vi "Manual_Override.vi"() -> ()   [LabVIEW 2020]
panel:
  out "error out":errorcluster
  in  "error in (no error)":errorcluster
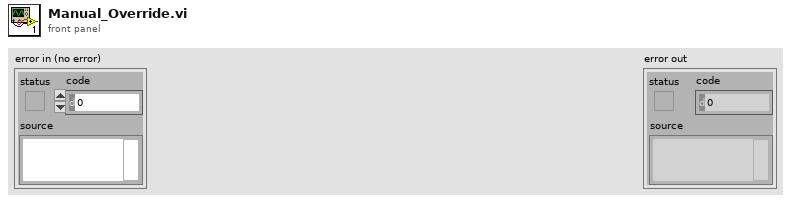
[diagram p1: front panel]
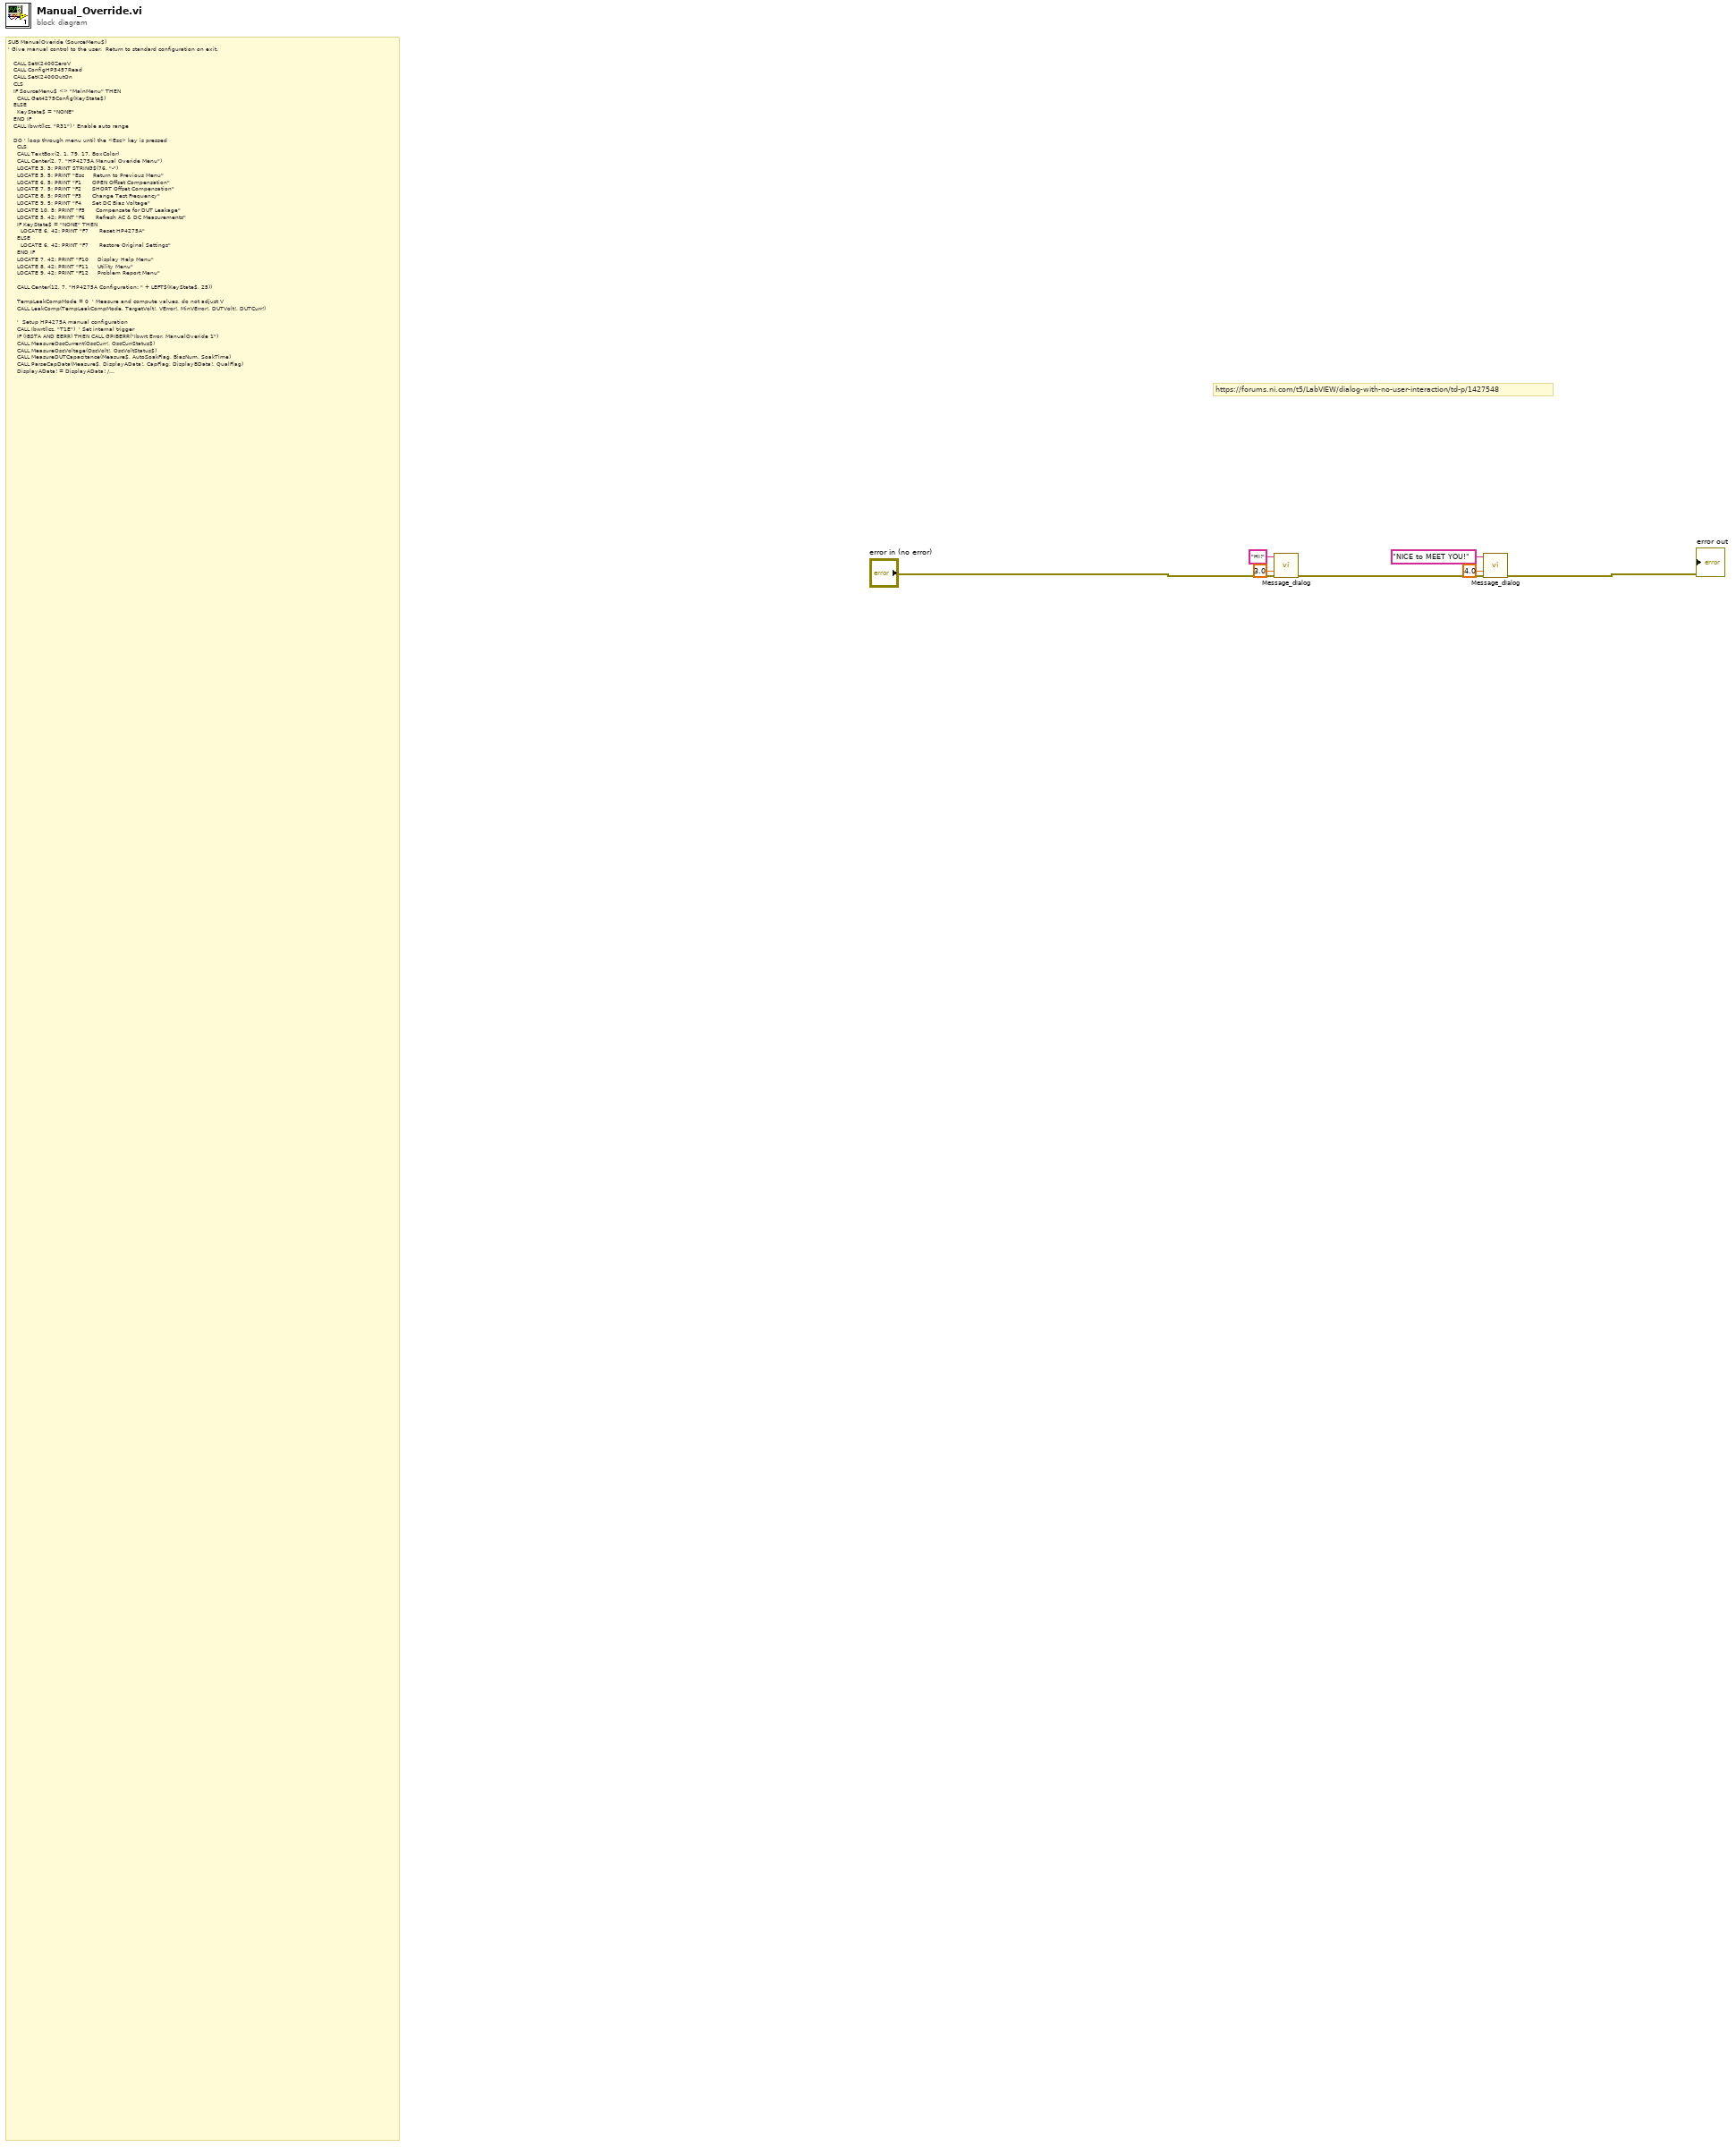
[diagram p0: block diagram]
diagram:
  # "https://forums.ni.com/t5/LabVIEW/dialog-with-no-user-interaction/td-p/1427548"
  # "SUB ManualOveride (SourceMenu$)\n' Give manual control to the user.  Return to standard configuration on exit.\n\n   CALL SetK2400ZeroV\n   CALL ConfigHP3457Read\n   CALL SetK2400OutOn\n   CLS\n   IF SourceMenu$ <> \"MainMenu\" THEN\n     CALL Get4275Config(KeyState$)\n   ELSE\n     KeyState$ = \"NONE\"\n   END IF\n   CALL Ibwrt(lcz, \"R31\") ' Enable auto range\n\n   DO ' loop through menu until the <Esc> key is pressed\n     CLS\n     CALL TextBox(2, 1, 79, 17, BoxColor)\n     CALL Center(2, 7, \"HP4275A Manual Overide Menu\")\n     LOCATE 3, 3: PRINT STRING$(76, \"-\")\n     LOCATE 5, 5: PRINT \"Esc     Return to Previous Menu\"\n     LOCATE 6, 5: PRINT \"F1      OPEN Offset Compensation\"\n     LOCATE 7, 5: PRINT \"F2      SHORT Offset Compensation\"\n     LOCATE 8, 5: PRINT \"F3      Change Test Frequency\"\n     LOCATE 9, 5: PRINT \"F4      Set DC Bias Voltage\"\n     LOCATE 10, 5: PRINT \"F5      Compensate for DUT Leakage\"\n     LOCATE 5, 42: PRINT \"F6      Refresh AC & DC Measurements\"\n     IF KeyState$ = \"NONE\" THEN\n       LOCATE 6, 42: PRINT \"F7      Reset HP4275A\"\n     ELSE\n       LOCATE 6, 42: PRINT \"F7      Restore Original Settings\"\n     END IF\n     LOCATE 7, 42: PRINT \"F10     Display Help Menu\"\n     LOCATE 8, 42: PRINT \"F11     Utility Menu\"\n     LOCATE 9, 42: PRINT \"F12     Problem Report Menu\"\n\n     CALL Center(12, 7, \"HP4275A Configuration: \" + LEFT$(KeyState$, 25))\n\n     TempLeakCompMode = 0  ' Measure and compute values, do not adjust V\n     CALL LeakComp(TempLeakCompMode, TargetVolt!, VError!, MinVError!, DUTVolt!, DUTCurr!)\n\n     '  Setup HP4275A manual configuration\n     CALL Ibwrt(lcz, \"T1E\")  ' Set internal trigger\n     IF (IBSTA AND EERR) THEN CALL GPIBERR(\"Ibwrt Error, ManualOveride 1\")\n     CALL MeasureOscCurrent(OscCurr!, OscCurrStatus$)\n     CALL MeasureOscVoltage(OscVolt!, OscVoltStatus$)\n     CALL MeasureDUTCapacitance(Measure$, AutoSoakFlag, BiasNum, SoakTime)\n     CALL ParseCapData(Measure$, DisplayAData!, CapFlag, DisplayBData!, QualFlag)\n     DisplayAData! = DisplayAData! / 1E+12\n     CALL IBLOC(lcz)\n\n     LOCATE 13, 5\n     PRINT \"Device DC Voltage:  \"; DUTVolt!; \"V\"\n     LOCATE 14, 5\n     PRINT \"Device DC Current:  \"; DUTCurr!; \"A\"\n     LOCATE 15, 5\n     PRINT \"Bias Voltage Error: \"; VError!\n     LOCATE 16, 5\n     PRINT \"Max Voltage Error:  \"; MaxVError!\n\n     LOCATE 13, 47\n     PRINT \"HP4275 Display A: \"; DisplayAData!;\n     LOCATE 14, 47\n     PRINT \"HP4275 Display B: \"; DisplayBData!;\n     LOCATE 15, 47\n     PRINT \"HP4275 Osc V:     \"; OscVolt!; \"V\"\n     LOCATE 16, 47\n     PRINT \"HP4275 Osc I:     \"; OscCurr!; \"A\"\n\n     CALL Center(18, 7, \"Ready\")\n\n     DO\n       Choice$ = INKEY$\n     LOOP WHILE Choice$ = \"\"\n     FOR x! = 1 TO 1000: z = RND: NEXT x!  'Keyboard read delay\n     DO   'Purge keyboard buffer\n       Temp$ = INKEY$\n     LOOP WHILE Temp$ <> \"\"\n\n     '  Convert 2-byte extended code to 1-byte ASCII code\n     Choice$ = RIGHT$(Choice$, 1)\n     SELECT CASE Choice$\n       CASE CHR$(F1)  ' OPEN Offset Compensation\n     CALL SetK2400ZeroV\n     CALL Delay(100)\n     CALL CalibrateOpen(TestLevel!, Flag, AutoSoakFlag)\n     CALL IBLOC(lcz)\n       CASE CHR$(F2)  ' SHORT Offset Compensation\n     CALL SetK2400ZeroV\n     CALL Delay(100)\n     CALL CalibrateShort(Flag, AutoSoakFlag)\n     CALL IBLOC(lcz)\n       CASE CHR$(F3)  ' Change Test Frequency\n     CALL SelectFreq(Flag)\n     CALL IBLOC(lcz)\n       CASE CHR$(F4)  ' Set DC Bias Voltage\n     LOCATE 18, 1: PRINT STRING$(76, \" \")\n     IF INSTR(UCASE$(VoltConfig$), \"H\") > 0 THEN\n       VoltMax! = 200!\n       VoltMin! = -200!\n     ELSE\n       VoltMax! = 35!\n       VoltMin! = -35!\n     END IF\n\n     PRINT \"  Enter bias voltage (\"; : PRINT USING \"####.#\"; VoltMin!;\n     PRINT \"V to\"; : PRINT USING \" +###.#\"; VoltMax!;\n     PRINT \"V).  Enter 999 to quit\";\n     INPUT Temp$\n     TempBias! = VAL(Temp$)\n     IF TempBias! <> 999! THEN\n       IF TempBias! > VoltMax! OR TempBias! < VoltMin! THEN\n         CALL SoundEff(2, 1)\n         PRINT\n         PRINT \"  Bias voltage must be between \";\n         PRINT USING \"####.#\"; VoltMin!;\n         PRINT \"V and \";\n         PRINT USING \"+###.#\"; VoltMax!;\n         PRINT \"V.\"\n         SLEEP 4: CALL SoundEff(2, 1)\n       ELSE\n         CALL SetK2400Voltage(TempBias!)\n         CALL Delay(300)\n         CALL MeasureDUTCurrent(DUTCurr!)\n       END IF\n     END IF\n       CASE CHR$(F5)  ' Compensate for DUT Leakage\n     LOCATE 18, 1: PRINT STRING$(76, \" \")\n     TargetVolt! = TempBias!\n     TempLeakCompMode = 1\n     CALL LeakComp(TempLeakCompMode, TargetVolt!, VError!, MinVError!, DUTVolt!, DUTCurr!)\n       CASE CHR$(F6)   ' Refresh AC & DC Measurements\n     ' Do nothing, measurements are updated every loop\n     LOCATE 18, 1: PRINT STRING$(76, \" \")\n       CASE CHR$(F7)  ' Reset HP4275A or Restore Original Settings\n     LOCATE 18, 1: PRINT STRING$(76, \" \")\n     CALL SetK2400ZeroV\n     IF KeyState$ = \"NONE\" THEN\n       CALL Ibclr(lcz)  ' Reset the HP4275A\n       CALL IBLOC(lcz)\n     ELSE\n       ' Restore original configuration\n       CALL Restore4275Config(KeyState$)\n       CALL Delay(100)\n       CALL Ibwrt(lcz, \"T1E\")  ' Set internal trigger\n       IF (IBSTA AND EERR) THEN CALL GPIBERR(\"Ibwrt Error, ManualOveride 2\")\n     END IF\n     CALL IBLOC(lcz)\n       CASE CHR$(F10)  ' Display Helpfile\n     CALL HelpMenu\n       CASE CHR$(F11)  ' Utility Menu\n     CALL UtilityMenu(SoakTime)\n       CASE CHR$(F12)  ' Problem Report Menu\n     ' Display report menu\n     CALL SelectReportType\n       CASE CHR$(Esc) ' Return to Previous Menu\n     LOCATE 18, 1: PRINT STRING$(76, \" \")\n       CASE ELSE\n     LOCATE 18, 1: PRINT STRING$(76, \" \")\n     LOCATE 18: PRINT \"      Invalid entry; returning to manual menu\"\n     CALL SoundEff(5, 1)\n     SLEEP 2\n     END SELECT\n   LOOP WHILE Choice$ <> CHR$(Esc)\n\n   CALL Center(18, 7, \"Returning to original configuration...\")\n   IF KeyState$ = \"NONE\" THEN\n     CALL Ibclr(lcz)  ' Reset the HP4275A\n     CALL IBLOC(lcz)\n   ELSE\n     ' Restore original configuration\n     CALL Ibwrt(lcz, KeyState$)\n     IF (IBSTA AND EERR) THEN CALL GPIBERR(\"Ibwrt Error, ManualOveride 3\")\n   END IF\n   CALL SetK2400ZeroV\n   SLEEP 1\n   CALL MeasureDUTVoltage(DUTVolt!) ' Refresh the HP3457 display\n   CALL ConfigHP3457Norm\n   CLS\n\nEND SUB"
  n1 = call "Message_dialog.vi"("error in (no error)"="error in (no error)", "set delay"=3.0, "String"="HI!") -> ("error out"=w6:errorcluster)  [unwired: 8 in]
  n2 = call "Message_dialog.vi"("error in (no error)"=w6, "set delay"=4.0, "String"="NICE to MEET YOU!") -> ("error out"=→"error out":errorcluster)  [unwired: 8 in]
